vi "Initialize.vi"(8 "error in (no error)":errorcluster, 9 "Reset (True)":bool=TRUE, 10 "ID Query (True)":bool=TRUE, 11 "VISA resource name":refnum<visa-resource-name>) -> (0 "error out":errorcluster, 3 "VISA resource name out":refnum<visa-resource-name>)   [LabVIEW 2023, in "Tektronix AFG 3000 Series.lvlib"]
doc: "Establishes communication with the instrument and optionally performs an instrument identification query and/or an instrument reset. It also places the instrument in a default state needed for other instrument driver operations. Therefore, call this VI before calling other instrument driver VIs for this instrument. Generally, you need to call the <B>Initialize VI</B> only once at the beginning of an application."
uses:
  Tektronix AFG 3000 Series.lvlib
panel:
  # "(c) 2006-2019 National Instruments.  ALL RIGHTS RESERVED."
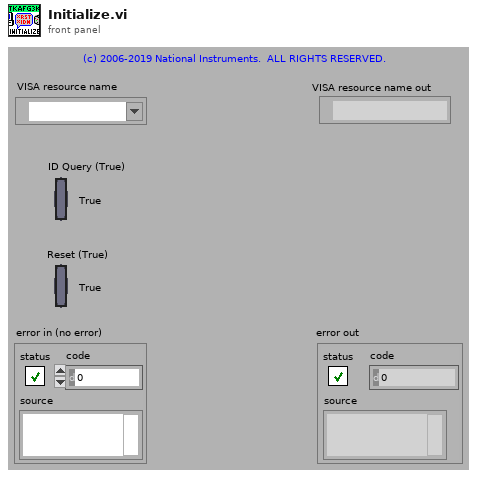
[diagram p1: front panel]
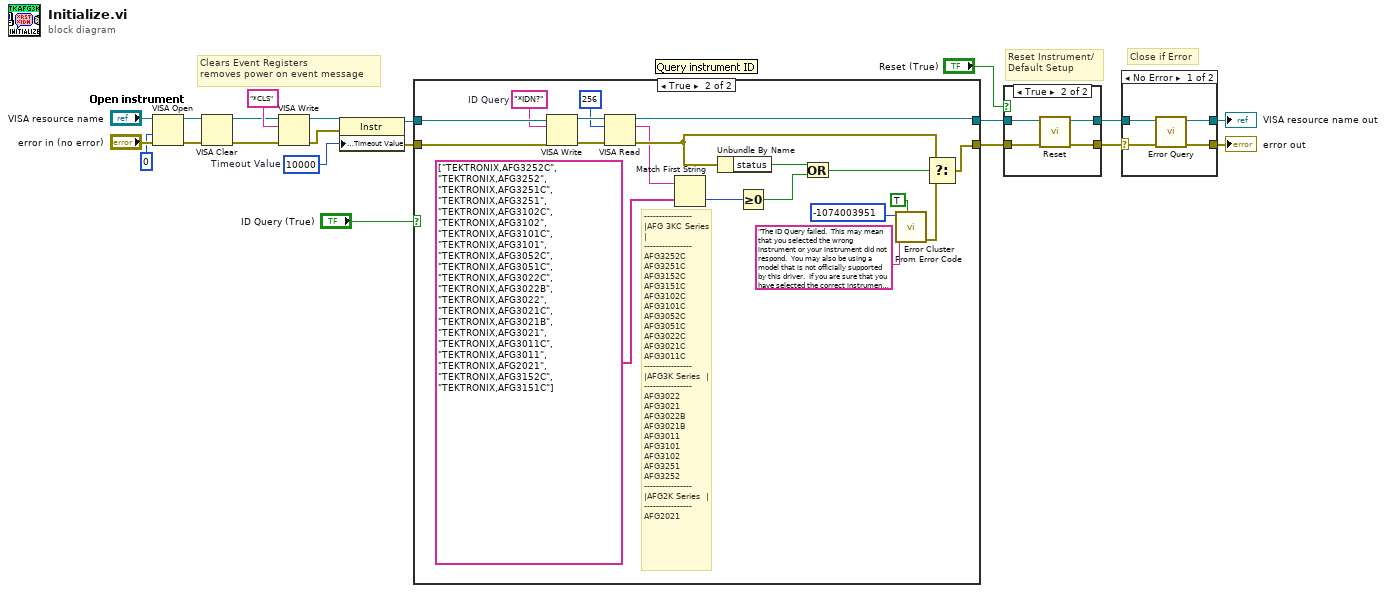
[diagram p0: block diagram]
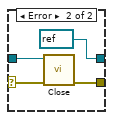
[diagram p2: hidden frame]
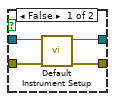
[diagram p3: hidden frame]
diagram:
  w6 = u32 10000  # Timeout Value
  # "Clears Event Registers \nremoves power on event message"
  # "Close if Error"
  # "Reset Instrument/\nDefault Setup"
  n1 = VISA Open(access mode=u32 0, error in (no error)="error in (no error)", VISA resource name="VISA resource name") -> (VISA resource name=w16:refnum<visa-resource-name>, error out=w15:errorcluster)  [unwired: 2 in]
  n2 = VISA Clear(VISA resource name=w16, error in (no error)=w15) -> (VISA resource name out=w4:refnum<visa-resource-name>, error out=w3:errorcluster)
  n3 = VISA Write(VISA resource name=w4, write buffer="*CLS", error in (no error)=w3) -> (VISA resource name out=w2:refnum<visa-resource-name>, error out=w1:errorcluster)  [unwired: 1 out]
  n4 = property class="Instr"(reference=w2, error in=w1, "General Settings:Timeout Value"=w6) -> (reference out=w8:refnum<visa-resource-name>, error out=w7:errorcluster)
  n5 = case shown="True" "ID Query (True)" {
    tunnel: [w22 w31] -> w9
    tunnel: [w23 w40] -> w10
    tunnel: w8 -> [w23 w41]
    tunnel: w7 -> [w22 w42]
    frame False {
    }
    frame True {
      w36 = "*IDN?"  # ID Query
      # "----------------\n|AFG 3KC Series |\n----------------\nAFG3252C\nAFG3251C\nAFG3152C\nAFG3151C\nAFG3102C\nAFG3101C\nAFG3052C\nAFG3051C\nAFG3022C\nAFG3021C\nAFG3011C\n----------------\n|AFG3K Series  |\n----------------\nAFG3022\nAFG3021\nAFG3022B\nAFG3021B\nAFG3011\nAFG3101\nAFG3102\nAFG3251\nAFG3252\n----------------\n|AFG2K Series  |\n----------------\nAFG2021"
      n6 = VISA Write(VISA resource name=w41, write buffer=w36, error in (no error)=w42) -> (VISA resource name out=w39:refnum<visa-resource-name>, error out=w38:errorcluster)  [unwired: 1 out]
      n7 = VISA Read(VISA resource name=w39, byte count=u32 256, error in (no error)=w38) -> (VISA resource name out=w40:refnum<visa-resource-name>, read buffer=w30:string, error out=w35:errorcluster)  [unwired: 1 out]
      n8 = Match First String(2:string[] ["TEKTRONIX,AFG3252C", "TEKTRONIX,AFG3252", "TEKTRONIX,AFG3251C", "TEKTRONIX,AFG3251", "TEKTRONIX,AFG3102C", "TEKTRONIX,AFG3102", "TEKTRONIX,AFG3101C", "TEKTRONIX,AFG3101", "TEKTRONIX,AFG3052C", "TEKTRONIX,AFG3051C", "TEKTRONIX,AFG3022C", "TEKTRONIX,AFG3022B", "TEKTRONIX,AFG3022", "TEKTRONIX,AFG3021C", "TEKTRONIX,AFG3021B", "TEKTRONIX,AFG3021", "TEKTRONIX,AFG3011C", "TEKTRONIX,AFG3011", "TEKTRONIX,AFG2021", "TEKTRONIX,AFG3152C", "TEKTRONIX,AFG3151C"] ("reversed array"), 3:w30) -> (0:w25:i32)  [unwired: 1 out]
      n9 = Unbundle By Name(w35) -> ("status"=w34:bool)
      n10 = Greater Or Equal To 0?(x=w25) -> (x >= 0?=w33:bool)
      n11 = Or(x=w34, y=w33) -> (x .or. y?=w32:bool)
      n12 = call <vilib>:"Error Cluster From Error Code.vi"("show call chain? (False)"=TRUE, "error message (\"\")"="The ID Query failed.  This may mean that you selected the wrong instrument or your instrument did not respond.  You may also be using a model that is not officially supported by this driver.  If you are sure that you have selected the correct instrument and it is responding, try disabling the ID Query." ("Source (VI Name)"), "error code (0)"=-1074003951 ("Code")) -> ("error out"=w26:errorcluster)  [unwired: 6 in]
      n13 = Select(t=w35, s=w32, f=w26) -> (s? t:f=w31:errorcluster)
    }
  }
  n14 = case shown="True" "Reset (True)" {
    tunnel: [w45 w50] -> w11
    tunnel: w10 -> [w46 w48]
    tunnel: [w44 w49] -> w12
    tunnel: w9 -> [w43 w47]
    frame False {
      n15 = call "Default Instrument Setup.vi"("error in (no error)"=w43, "VISA resource name"=w46) -> ("error out"=w45:errorcluster, "VISA resource name out"=w44:refnum<visa-resource-name>)  [unwired: 8 in]
    }
    frame True {
      n16 = call "Reset.vi"("error in (no error)"=w47, "VISA resource name"=w48) -> ("error out"=w50:errorcluster, "VISA resource name out"=w49:refnum<visa-resource-name>)  [unwired: 8 in]
    }
  }
  n17 = case shown="No Error" w11 {
    selector: w11 -> [w52 w56]
    tunnel: w12 -> [w51 w57]
    tunnel: [w54 refnum<visa-resource-name> refnum ("VISA resource name out")] -> w14
    tunnel: [w53 w58] -> w13
    frame No Error {
      n18 = call "Error Query.vi"("error in (no error)"=w52, "VISA resource name"=w51) -> ("error out"=w53:errorcluster, "VISA resource name out"=w54:refnum<visa-resource-name>)  [unwired: 6 in, 2 out]
    }
    frame Error {
      n19 = call "Close.vi"("error in (no error)"=w56, "VISA resource name"=w57) -> ("error out"=w58:errorcluster)  [unwired: 9 in]
    }
  }
  "VISA resource name out" <- w14
  "error out" <- w13
